vi "Read Discrete Inputs.vi"(7 "unit ID":u8, 8 "error in":errorcluster, 9 "number of inputs":u16, 10 "starting address":u16, 11 "Modbus slave in":refnum<class "Modbus Slave.lvclass">) -> (0 "error out":errorcluster, 2 "discrete inputs":bool[](array[boolean]), 3 "Modbus slave out":refnum<class "Modbus Slave.lvclass">)   [LabVIEW 2013, in "Modbus Library - Advance.lvlib" / "Modbus Slave.lvclass"]
doc: "Reads <B>number of inputs</B> discrete inputs starting at <B>starting address</B> from the device."
uses:
  Modbus Slave.lvclass
  Modbus Slave.lvclass/Modbus Slave.ctl
  Standard Data Model/Standard Data Model.lvclass
  Super Data Model/Super Data Model.lvclass
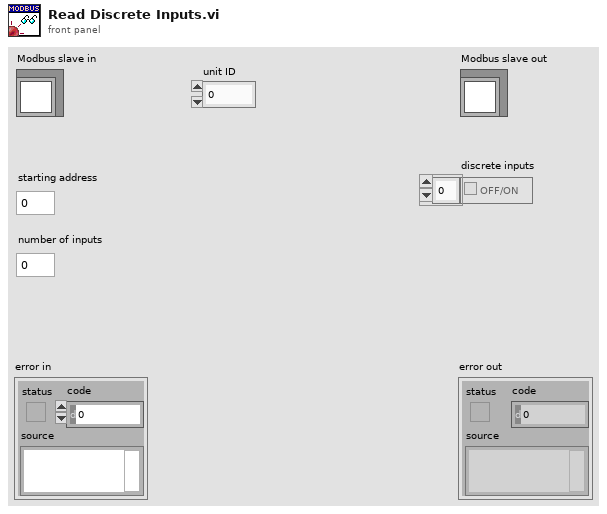
[diagram p1: front panel]
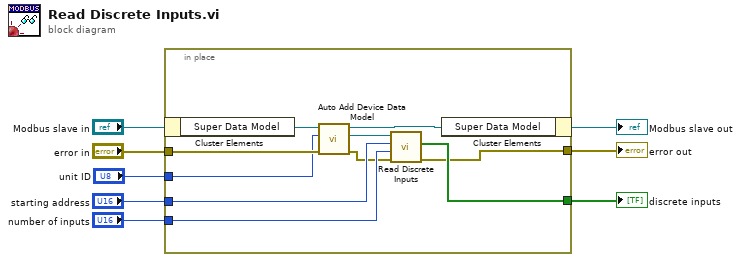
[diagram p0: block diagram]
diagram:
  n1 = in-place {
    in-place-border: [w18] -> w6
    in-place-border: "number of inputs" -> [w17]
    in-place-border: "starting address" -> [w16]
    in-place-border: [w15] -> w3
    in-place-border: "error in" -> [w13]
    in-place-border: "unit ID" -> [w9]
    n2 = in-place-cluster #1("Modbus slave in") -> ("Super Data Model"=w14:refnum<class "Super Data Model.lvclass">)
    n3 = call "Auto Add Device Data Model.vi"("error in"=w13, "unit ID"=w9, "Super Data Model in"=w14) -> ("error out"=w12:errorcluster, "device data model"=w11:refnum<class "Standard Data Model.lvclass">, "Super Data Model out"=w10:refnum<class "Super Data Model.lvclass">)  [unwired: 6 in]
    n4 = call-dynamic "Read Discrete Inputs.vi"("error in"=w12, "number of inputs"=w17, "starting address"=w16, "device data model in"=w11) -> ("error out"=w15:errorcluster, "data"=w18:bool[])  [unwired: 5 in, 1 out]
    n5 = in-place-cluster #1("Super Data Model"=w10) -> (→"Modbus slave out":refnum<class "Modbus Slave.lvclass">)
  }
  "error out" <- w3
  "discrete inputs" <- w6
